vi "LR700_talk.vi"(8 "error in":errorcluster, 10 "Send":string, 11 "Address":i32) -> (0 "error out":errorcluster, 3 "read":string="\n")   [LabVIEW 2014]
panel:
  in  "mode (0) 2":i16=32
  in  "mode (0)":i16=3
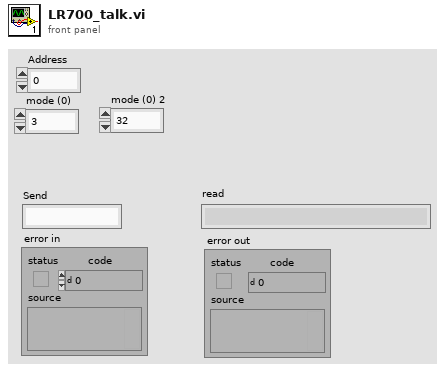
[diagram p1: front panel]
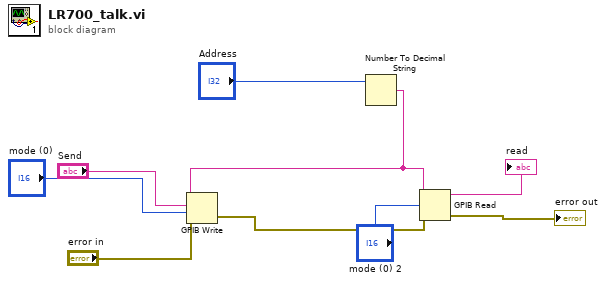
[diagram p0: block diagram]
diagram:
  n1 = Number To Decimal String(number="Address") -> (decimal integer string=w2:string)  [unwired: 1 in]
  n2 = GPIB Write(0:w2, 1:"Send", 2:"mode (0)", 3:"error in") -> (6:w9:errorcluster)  [unwired: 1 in, 1 out]
  n3 = GPIB Read(0:w2, 1:"mode (0) 2", 3:w9) -> (5:→"read":string, 7:→"error out":errorcluster)  [unwired: 2 in, 1 out]
